vi "Direttore.read.fpga.vi"   [LabVIEW 2012]
uses:
  <vilib>/rvi/interface/RandomDataEmulation/nirviRandomDataFPGAFIFO.vi
  <vilib>/rvi/interface/RandomDataEmulation/niFpgaRandomDataHandleErrors.vi
  <vilib>/rvi/DataTransferAndStorage/Container/XNode/niFpgaContainer.xnode
  <vilib>/rvi/interface/RandomDataEmulation/nirviRandomDataFpgaReadWriteTemplate.vi
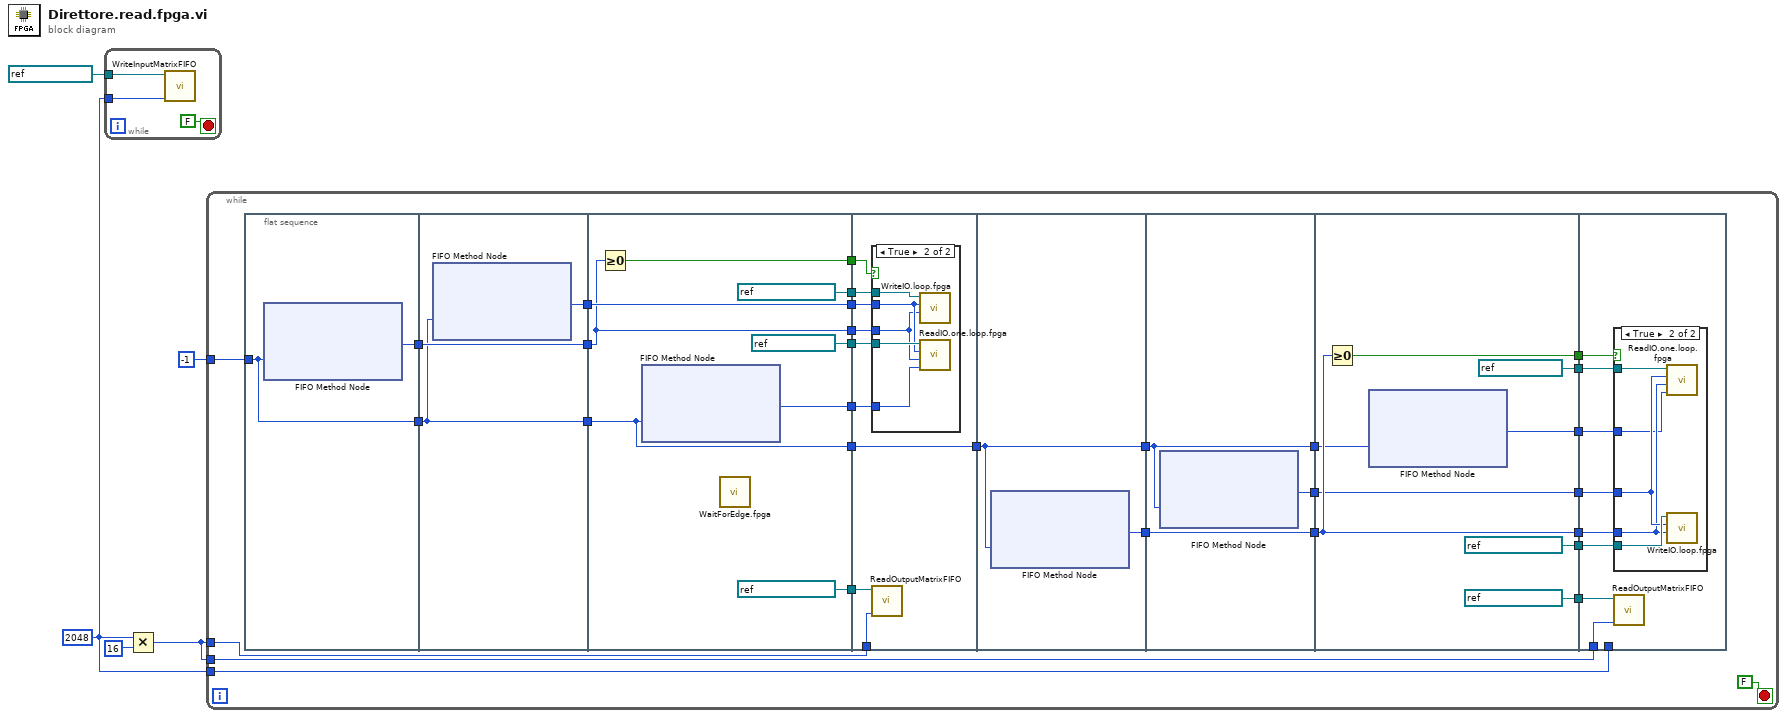
[diagram p0: block diagram]
diagram:
  w1 = 2048
  n1 = while {
    tunnel: w1 -> [w6]
    tunnel: refnum<k21> "InputMatrix" ("Memory In") -> [w7]
    stop <- FALSE stop-if-true
    n2 = call "WriteInputMatrixFIFO.vi"("Matrix length (in)"=w6, "Memory In"=w7) -> ()  [unwired: 10 in]
  }
  n3 = Multiply(x=w1, y=16 ("Numeric")) -> (x*y=w4:i32)
  n4 = while {
    tunnel: w1 -> [w39]
    tunnel: w4 -> [w37]
    tunnel: w4 -> [w36]
    tunnel: -1 ("Timeout") -> [w23]
    stop <- FALSE stop-if-true
    n5 = flat-sequence {
      tunnel: w23 -> [w41]
      tunnel: [w41] -> w18
      tunnel: [w40] -> w16
      tunnel: [w42] -> w19
      tunnel: w18 -> [w43]
      tunnel: [w43] -> w17
      tunnel: w16 -> [w44]
      tunnel: [w44] -> w15
      tunnel: [w52] -> w35
      tunnel: [w45] -> w34
      tunnel: [refnum<k21> "OutputMatrix1" ("Memory In")] -> w29
      tunnel: [refnum<k21> "InputMatrix" ("Memory (in)")] -> w28
      tunnel: [refnum<k21> "OutputMatrix2" ("Memory (in)")] -> w27
      tunnel: [w48] -> w26
      tunnel: [w47] -> w24
      tunnel: [w46] -> w22
      tunnel: w19 -> [w52]
      tunnel: w17 -> [w47]
      tunnel: w15 -> [w45]
      tunnel: w35 -> [w59]
      tunnel: w34 -> [w60]
      tunnel: w37 -> [w61]
      tunnel: w29 -> [w58]
      tunnel: w28 -> [w57]
      tunnel: w27 -> [w56]
      tunnel: w26 -> [w55]
      tunnel: w24 -> [w54]
      tunnel: [w54] -> w20
      tunnel: w22 -> [w53]
      tunnel: w20 -> [w67]
      tunnel: [w68] -> w14
      tunnel: [w67] -> w12
      tunnel: w14 -> [w70]
      tunnel: [w70] -> w13
      tunnel: w12 -> [w71]
      tunnel: [w71] -> w11
      tunnel: [w69] -> w9
      tunnel: [w74] -> w33
      tunnel: [refnum<k21> "OutputMatrix2" ("Memory In")] -> w32
      tunnel: [refnum<k21> "OutputMatrix1" ("Memory (in)")] -> w31
      tunnel: [refnum<k21> "InputMatrix" ("Memory (in)")] -> w30
      tunnel: [w76] -> w25
      tunnel: [w75] -> w21
      tunnel: w13 -> [w74]
      tunnel: w11 -> [w73]
      tunnel: [w72] -> w10
      tunnel: w9 -> [w72]
      tunnel: w33 -> [w87]
      tunnel: w39 -> [_]
      tunnel: w36 -> [w86]
      tunnel: w32 -> [w85]
      tunnel: w31 -> [w84]
      tunnel: w30 -> [w83]
      tunnel: w25 -> [w82]
      tunnel: w21 -> [w81]
      tunnel: w10 -> [w80]
      frame #0 {
        n6 = xnode ("FIFO Method Node")("Timeout"=w41) -> ("Element"=w40:i16)  [unwired: 1 in, 2 out]
      }
      frame #1 {
        n7 = xnode ("FIFO Method Node")("Timeout"=w43) -> ("Element"=w42:i16)  [unwired: 1 in, 2 out]
      }
      frame #2 {
        n8 = Greater Or Equal To 0?(x=w45) -> (x >= 0?=w48:bool)
        n9 = xnode ("FIFO Method Node")("Timeout"=w47) -> ("Element"=w46:i16)  [unwired: 1 in, 2 out]
        n10 = call "WaitForEdge.fpga.vi"() -> ()  [unwired: 12 in]
      }
      frame #3 {
        n11 = case shown="True" w55 {
          tunnel: w59 -> [_ w64]
          tunnel: w60 -> [_ w63]
          tunnel: w57 -> [_ w65]
          tunnel: w56 -> [_ w66]
          tunnel: w53 -> [_ w62]
          frame False {
          }
          frame True {
            n12 = call "WriteIO.loop.fpga.vi"("Delta time"=w63, "Number of time points"=w64, "Memory (in)"=w66) -> ()  [unwired: 9 in]
            n13 = call "ReadIO.one.loop.fpga.vi"("Channel"=w62, "Delta time"=w63, "Number of time points"=w64, "Memory (in)"=w65) -> ()  [unwired: 8 in]
          }
        }
        n14 = call "ReadOutputMatrixFIFO.vi"("Matrix length (in)"=w61, "Memory In"=w58) -> ()  [unwired: 10 in]
      }
      frame #4 {
        n15 = xnode ("FIFO Method Node")("Timeout"=w67) -> ("Element"=w68:i16)  [unwired: 1 in, 2 out]
      }
      frame #5 {
        n16 = xnode ("FIFO Method Node")("Timeout"=w71) -> ("Element"=w69:i16)  [unwired: 1 in, 2 out]
      }
      frame #6 {
        n17 = Greater Or Equal To 0?(x=w74) -> (x >= 0?=w76:bool)
        n18 = xnode ("FIFO Method Node")("Timeout"=w73) -> ("Element"=w75:i16)  [unwired: 1 in, 2 out]
      }
      frame #7 {
        n19 = case shown="True" w82 {
          tunnel: w87 -> [_ w89]
          tunnel: w80 -> [_ w90]
          tunnel: w84 -> [_ w92]
          tunnel: w83 -> [_ w91]
          tunnel: w81 -> [_ w88]
          frame False {
          }
          frame True {
            n20 = call "ReadIO.one.loop.fpga.vi"("Channel"=w88, "Delta time"=w89, "Number of time points"=w90, "Memory (in)"=w91) -> ()  [unwired: 8 in]
            n21 = call "WriteIO.loop.fpga.vi"("Delta time"=w89, "Number of time points"=w90, "Memory (in)"=w92) -> ()  [unwired: 9 in]
          }
        }
        n22 = call "ReadOutputMatrixFIFO.vi"("Matrix length (in)"=w86, "Memory In"=w85) -> ()  [unwired: 10 in]
      }
    }
  }
